vi "Check Time Error.vi"(8 "error in (no error)":errorcluster) -> (0 "error out":errorcluster, 3 "successful actuation?":bool)   [LabVIEW 2020, in "DAQmx Servo.lvclass"]
uses:
  DAQmx Servo.lvclass
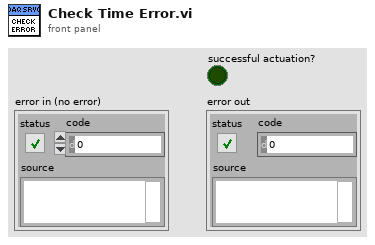
[diagram p1: front panel]
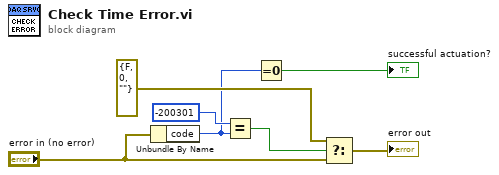
[diagram p0: block diagram]
diagram:
  n1 = Unbundle By Name("error in (no error)") -> ("code"=w2:i32)
  n2 = Equal?(x=-200301, y=w2) -> (x = y?=w6:bool)
  n3 = Equal To 0?(x=w2) -> (x = 0?=→"successful actuation?":bool)
  n4 = Select(t=errorcluster {"status"=FALSE, "code"=0, "source"=""}, s=w6, f="error in (no error)") -> (s? t:f=→"error out":errorcluster)
